vi "getGaussianArray.vi"(0 "#samples":u32, 1 "tiempo (ms)":u32, 2 "t0 (ms)":dbl, 3 "Sigma (ms)":dbl, 4 "Amplitud":dbl) -> (5 "Y out":dbl[](array[numeric]), 6 "t out":sgl[](array[numeric]))   [LabVIEW 2010]
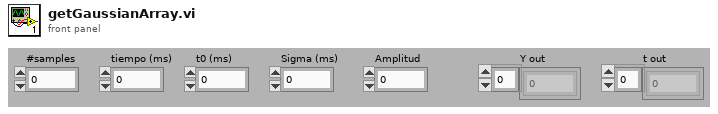
[diagram p1: front panel]
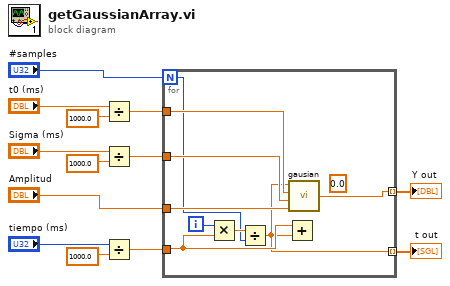
[diagram p0: block diagram]
diagram:
  n1 = Divide(x="t0 (ms)", y=sgl 1000.0) -> (x/y=w9:dbl)
  n2 = Divide(x="Sigma (ms)", y=sgl 1000.0) -> (x/y=w10:dbl)
  n3 = Divide(x="tiempo (ms)", y=sgl 1000.0) -> (x/y=w1:sgl)
  n4 = for {
    N: "#samples" -> [w18]
    tunnel: [w14] -> w11 mode=indexing
    tunnel: "Amplitud" -> [w21]
    tunnel: w10 -> [w20]
    tunnel: w9 -> [w19]
    tunnel: w1 -> [w16]
    tunnel: [w15] -> w13 mode=indexing
    i -> [w17]
    (unwired) 0.0 ("x")
    n5 = Multiply(x=w17, y=w16) -> (x*y=w22:sgl)
    n6 = Divide(x=w22, y=w18) -> (x/y=w15:sgl)
    n7 = Add(x=w16, y=w15) -> ()  [unwired: 1 out]
    n8 = call "gausian.vi"("Amplitud"=w21, "sigma"=w20, "miu"=w19, "x"=w15) -> ("out"=w14:dbl)
  }
  "t out" <- w13
  "Y out" <- w11
